vi "StartCandidateCSMs.vi"(8 "error in (no error)":errorcluster, 11 "TestCase in":refnum<class "testcase-CSMChainMode.lvclass">) -> (0 "error out":errorcluster, 3 "TestCase out":refnum<class "testcase-CSMChainMode.lvclass">)   [LabVIEW 2017, in "testcase-CSMChainMode.lvclass"]
uses:
  testcase-CSMChainMode.lvclass
  testcase-CSMChainMode.lvclass/testcase-CSMChainMode.ctl
  CSM/Chain4.vi
  CSM/Chain5.vi
  CSM/Chain6.vi
  <vilib>/addons/_JKI Toolkits/VI Tester/TestCase.llb/TestCase.lvclass
  src/user.lib/_NEVSTOP/Communicable State Machine(CSM)/Communicable State Machine.lvlib
  CSM/CSM-Testcase.lvlib
  C:/Program Files (x86)/National Instruments/LabVIEW 2017/vi.lib/addons/_JKI Toolkits/VI Tester/TestCase.llb/TestCase.lvclass
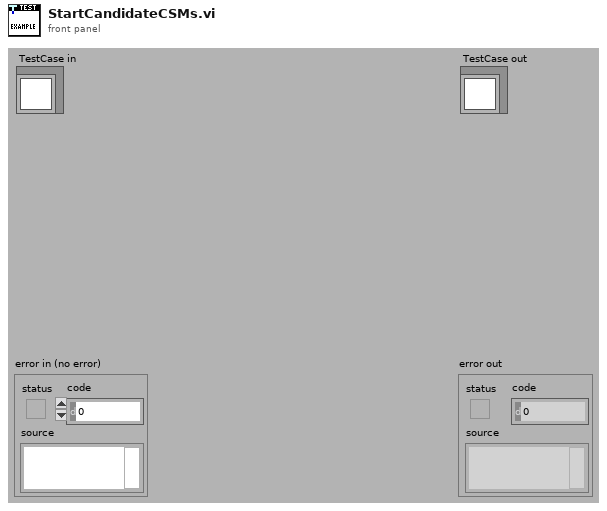
[diagram p1: front panel]
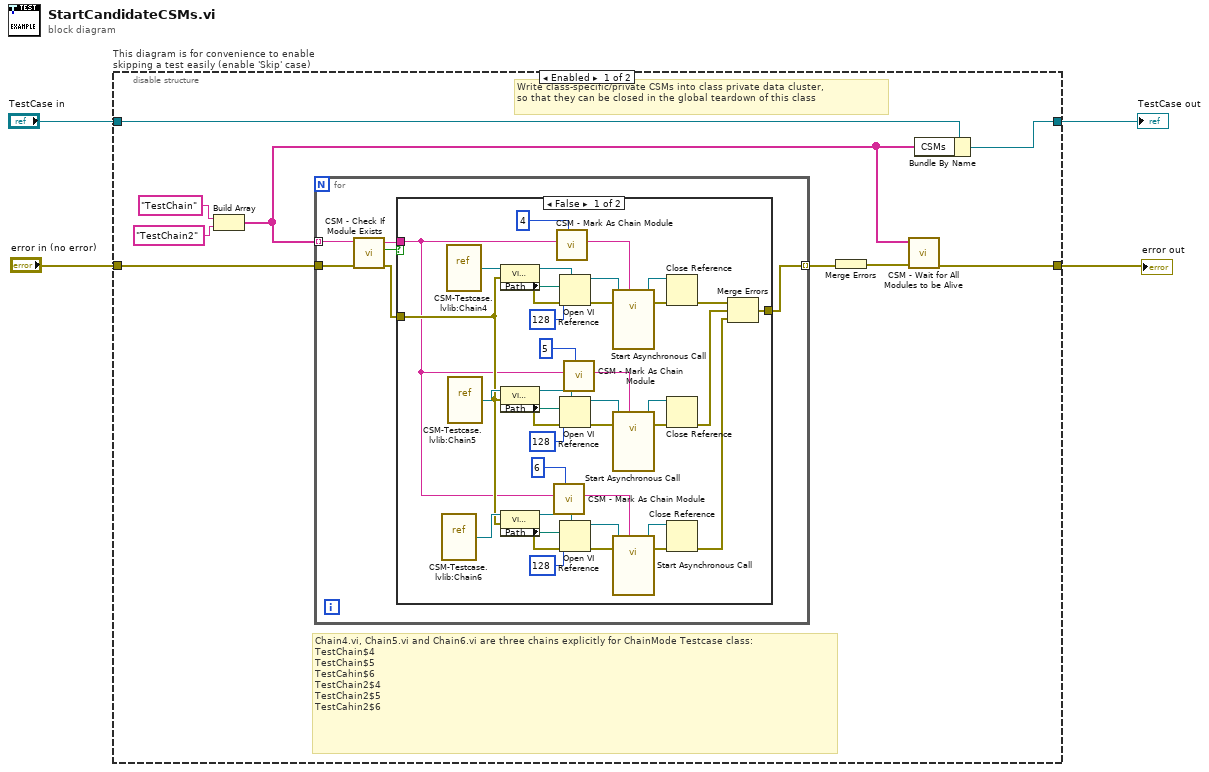
[diagram p0: block diagram]
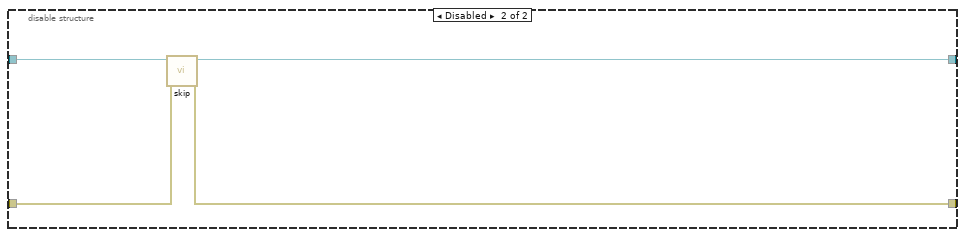
[diagram p3: hidden frame]
diagram:
  n1 = disable-structure "This diagram is for convenience to enable skipping a test easily (enable 'Skip' case)" shown="Enabled" {
    disable-tunnel: "TestCase in" -> [w13 w63]
    disable-tunnel: [w12 w61] -> w1
    disable-tunnel: [w10 w62] -> w3
    disable-tunnel: "error in (no error)" -> [w11 w60]
    frame Enabled {
      # "Write class-specific/private CSMs into class private data cluster,\nso that they can be closed in the global teardown of this class"
      # "Chain4.vi, Chain5.vi and Chain6.vi are three chains explicitly for ChainMode Testcase class:\nTestChain$4\nTestChain$5\nTestCahin$6\nTestChain2$4\nTestChain2$5\nTestCahin2$6"
      n2 = Build Array("TestChain" ("CSM Name"), "TestChain2" ("CSM Name")) -> (w7:string[])
      n3 = for {
        tunnel: w7 -> [w16] mode=indexing
        tunnel: w11 -> [w15]
        tunnel: [w14] -> w6 mode=indexing
        n4 = call "CSM - Check If Module Exists.vi"("Error In"=w15, "CSM Name"=w16) -> ("error out"=w17:errorcluster, "Exist?"=w19:bool, "CSM Name (Dup)"=w18:string)  [unwired: 7 in]
        n5 = case shown="False" w19 {
          tunnel: [w22 w59] -> w14
          tunnel: w17 -> [w21 w59]
          tunnel: w18 -> [w20 _]
          frame False {
            n6 = vi-ref "CSM-Testcase.lvlib:Chain6.vi"() -> (w40:refnum<vi>)
            n7 = vi-ref "CSM-Testcase.lvlib:Chain4.vi"() -> (w58:refnum<vi>)
            n8 = vi-ref "CSM-Testcase.lvlib:Chain5.vi"() -> (w41:refnum<vi>)
            n9 = property class="VI (strict)"(reference=w58, error in=w21) -> (reference out=w55:refnum<vi>, error out=w53:errorcluster, "Path"=w52:path)
            n10 = property class="VI (strict)"(reference=w41, error in=w21) -> (reference out=w44:refnum<vi>, error out=w46:errorcluster, "Path"=w47:path)
            n11 = property class="VI (strict)"(reference=w40, error in=w21) -> (reference out=w37:refnum<vi>, error out=w35:errorcluster, "Path"=w34:path)
            n12 = call "CSM - Mark As Chain Module.vi"("Order"=6, "CSM Name"=w20) -> ("CSM Name (Marked As Chain)"=w28:string)  [unwired: 8 in]
            n13 = call "CSM - Mark As Chain Module.vi"("Order"=4, "CSM Name"=w20) -> ("CSM Name (Marked As Chain)"=w26:string)  [unwired: 8 in]
            n14 = Open VI Reference(type specifier VI Refnum (for type only)=w55, vi path=w52, options=128, error in (no error)=w53) -> (vi reference=w51:refnum<vi>, error out=w56:errorcluster)  [unwired: 2 in]
            n15 = Open VI Reference(type specifier VI Refnum (for type only)=w44, vi path=w47, options=128, error in (no error)=w46) -> (vi reference=w48:refnum<vi>, error out=w43:errorcluster)  [unwired: 2 in]
            n16 = Open VI Reference(type specifier VI Refnum (for type only)=w37, vi path=w34, options=128, error in (no error)=w35) -> (vi reference=w33:refnum<vi>, error out=w38:errorcluster)  [unwired: 2 in]
            n17 = call "CSM - Mark As Chain Module.vi"("Order"=5, "CSM Name"=w20) -> ("CSM Name (Marked As Chain)"=w27:string)  [unwired: 8 in]
            n18 = call-by-ref "Start Asynchronous Call"(reference=w51, error in=w56, "Name (\"\" to Use UUID)"=w26) -> (reference out=w50:refnum<vi>, error out=w54:errorcluster)  [unwired: 11 in]
            n19 = call-by-ref "Start Asynchronous Call"(reference=w48, error in=w43, "Name (\"\" to Use UUID)"=w27) -> (reference out=w49:refnum<vi>, error out=w45:errorcluster)  [unwired: 11 in]
            n20 = call-by-ref "Start Asynchronous Call"(reference=w33, error in=w38, "Name (\"\" to Use UUID)"=w28) -> (reference out=w32:refnum<vi>, error out=w36:errorcluster)  [unwired: 11 in]
            n21 = Close Reference(reference=w50, error in (no error)=w54) -> (error out=w31:errorcluster)
            n22 = Close Reference(reference=w49, error in (no error)=w45) -> (error out=w30:errorcluster)
            n23 = Close Reference(reference=w32, error in (no error)=w36) -> (error out=w29:errorcluster)
            n24 = Merge Errors(w31, w30, w29) -> (w22:errorcluster)
          }
          frame True {
          }
        }
      }
      n25 = Merge Errors(w6) -> (w5:errorcluster)
      n26 = call "CSM - Wait for All Modules to be Alive.vi"("Error In"=w5, "CSM Names"=w7) -> ("error out"=w10:errorcluster)  [unwired: 7 in, 2 out]
      n27 = Bundle By Name(cluster=w13, "CSMs"=w7) -> (w12:refnum<class "testcase-CSMChainMode.lvclass">)
    }
    frame Disabled {
      # "skip test result while test is under development"
      n28 = call <vilib>:"skip.vi"("error in (no error)"=w60, "TestCase in"=w63) -> ("error out"=w62:errorcluster, "TestCase out"=w61:refnum<class "testcase-CSMChainMode.lvclass">)  [unwired: 8 in]
    }
  }
  "error out" <- w3
  "TestCase out" <- w1
